vi "SaveTemp.vi"(10 "new name":string, 11 "Original":path) -> (0 "error out":errorcluster, 3 "temporary":path)   [LabVIEW 2022 SP3]
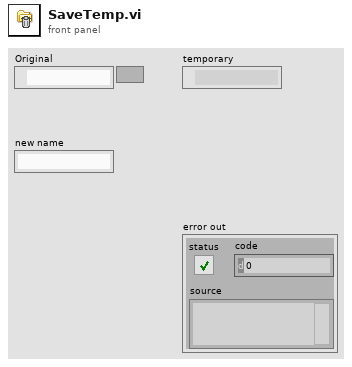
[diagram p1: front panel]
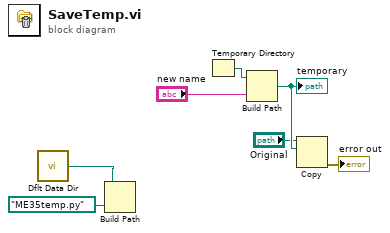
[diagram p0: block diagram]
diagram:
  n1 = call <vilib>:"Dflt Data Dir.vi"() -> ("App:Default Data Directory"=w2:path)
  n2 = Build Path(base path=w2, name or relative path=path "ME35temp.py") -> ()  [unwired: 1 out]
  n3 = Temporary Directory() -> (w3:path)
  n4 = Build Path(base path=w3, name or relative path="new name") -> (appended path=w7:path)
  "temporary" <- w7
  n5 = Copy(10:w7, 11:"Original") -> (0:→"error out":errorcluster)  [unwired: 3 in, 2 out]
